vi "taskqueue ref.vi"(8 "错误输入（无错误）":errorcluster) -> (0 "错误输出":errorcluster, 3 "队列输出":refnum<queue>)   [LabVIEW 2016, in "斯坦道原位多参数.lvlib"]
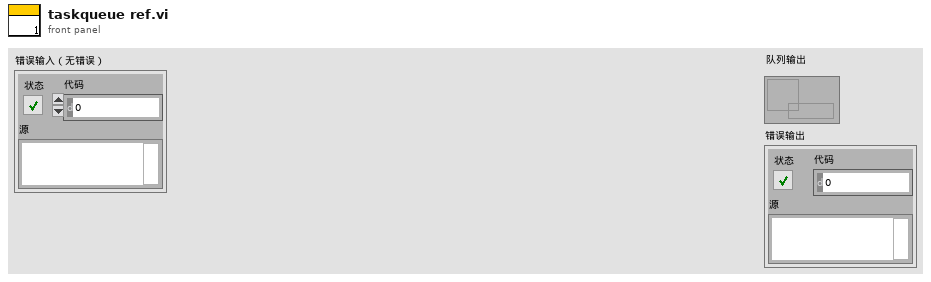
[diagram p1: front panel]
types:
  T1 = typedef "斯坦道原位多参数.lvlib/水样测试启动自定义输入参数.ctl" = cluster{"测量模式":string, "数据类型":string}
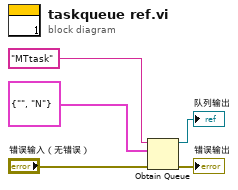
[diagram p0: block diagram]
diagram:
  n1 = Obtain Queue(name (unnamed)="MTtask" ("名称（未命名）"), element data type=T1 {"测量模式"="", "数据类型"="N"} ("启动参数"), error in (no error)="错误输入（无错误）") -> (queue out=→"队列输出":refnum<queue>, error out=→"错误输出":errorcluster)  [unwired: 2 in, 1 out]
